vi "Control multiple valves.vi"() -> ()   [LabVIEW 2016]
uses:
  Classes/Controller/I-O/NI-DAQ Folder/NI-DAQ.lvclass
panel:
  in  "stop":bool
  out "subarray":bool[](array[boolean])
  in  "Values":bool[](array[boolean])
  in  "Indices":i32[](array[numeric])
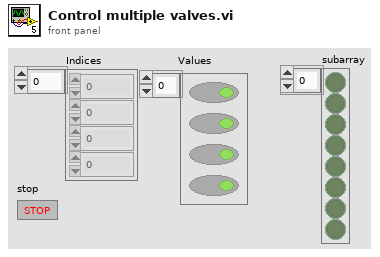
[diagram p1: front panel]
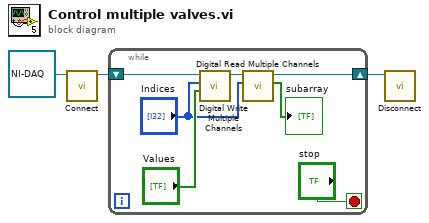
[diagram p0: block diagram]
diagram:
  n1 = call-dynamic "Connect.vi"("NI-DAQ in"=refnum<class "NI-DAQ.lvclass"> refnum ("NI-DAQ.lvclass")) -> ("NI-DAQ out"=w2:refnum<class "NI-DAQ.lvclass">)  [unwired: 9 in, 1 out]
  n2 = while {
    shift-right: [w6] -> w1
    shift-left: w2 -> [w10]
    stop <- "stop" stop-if-true
    n3 = call-dynamic "Digital Write Multiple Channels.vi"("Values"="Values", "Indices"="Indices", "NI-DAQ in"=w10) -> ("NI-DAQ out"=w9:refnum<class "NI-DAQ.lvclass">)  [unwired: 7 in, 1 out]
    n4 = call-dynamic "Digital Read Multiple Channels.vi"("Array"="Indices", "NI-DAQ in"=w9) -> ("subarray"=→"subarray":bool[], "NI-DAQ out"=w6:refnum<class "NI-DAQ.lvclass">)  [unwired: 7 in, 1 out]
  }
  n5 = call-dynamic "Disconnect.vi"("I-O in"=w1) -> ()  [unwired: 9 in, 1 out]
